vi "实时数据参数入列队.vi"(11 "发送实时数据选择框":T1) -> (0 "错误输出":errorcluster)   [LabVIEW 2016]
panel:
  out "数组":string[](array[string])
  # "水样测量"
  # "零点核查"
  # "跨度核查"
  # "加标回收"
  # "平行样"
  # "标样核查"
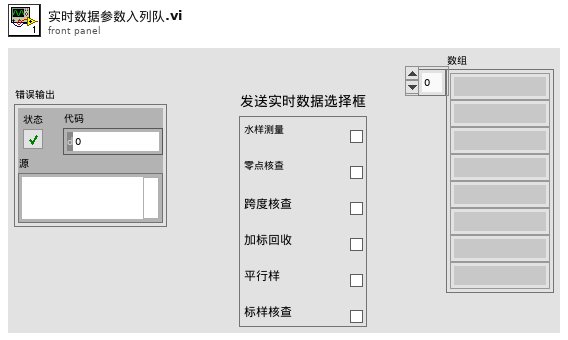
[diagram p1: front panel]
types:
  T1 = cluster{"水样测试":bool, "空白测试":bool, "跨度核查":bool, "加标回收":bool, "平行样":bool, "标样核查":bool}
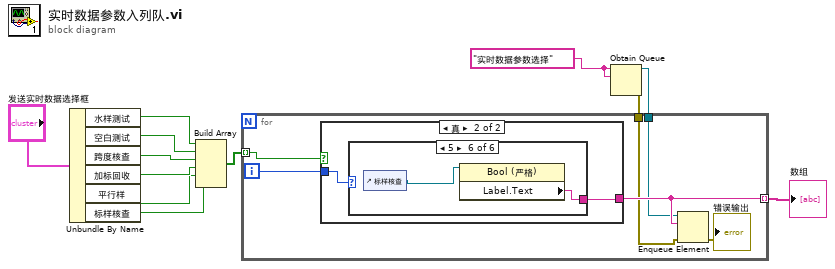
[diagram p0: block diagram]
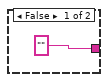
[diagram p2: hidden frame]
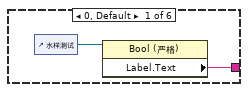
[diagram p3: hidden frame]
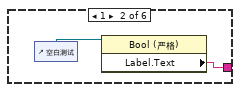
[diagram p4: hidden frame]
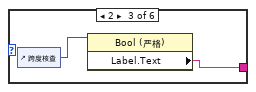
[diagram p5: hidden frame]
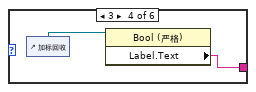
[diagram p6: hidden frame]
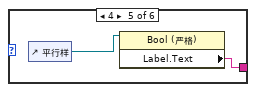
[diagram p7: hidden frame]
diagram:
  w3 = "实时数据参数选择" ("名称（未命名）")
  n1 = Unbundle By Name("发送实时数据选择框") -> ("水样测试"=w11:bool, "空白测试"=w10:bool, "跨度核查"=w9:bool, "加标回收"=w8:bool, "平行样"=w7:bool, "标样核查"=w1:bool)
  n2 = Build Array(w11, w10, w9, w8, w7, w1) -> (w6:bool[])
  n3 = Obtain Queue(name (unnamed)=w3, element data type=w3) -> (queue out=w4:refnum<queue>, error out=w2:errorcluster)  [unwired: 3 in, 1 out]
  n4 = for {
    tunnel: w6 -> [w18] mode=indexing
    tunnel: [w16] -> w5 mode=indexing
    tunnel: w4 -> [w15]
    tunnel: w2 -> [w14]
    i -> [w17]
    n5 = case shown="真" w18 {
      tunnel: w17 -> [_ w21]
      tunnel: ["" ("Label.Text") w20] -> w16
      frame False {
      }
      frame True {
        n6 = case shown="5" w21 {
          tunnel: [w22 w24 w27 w28 w30 w33] -> w20
          frame 0, Default {
            n7 = control-ref of="水样测试"() -> (w23:refnum<vi>)
            n8 = property class="Bool (严格)"(reference=w23) -> ("Label.Text"=w22:string)  [unwired: 1 in, 2 out]
          }
          frame 1 {
            n9 = control-ref of="空白测试"() -> (w25:refnum<vi>)
            n10 = property class="Bool (严格)"(reference=w25) -> ("Label.Text"=w24:string)  [unwired: 1 in, 2 out]
          }
          frame 2 {
            n11 = control-ref of="跨度核查"() -> (w26:refnum<vi>)
            n12 = property class="Bool (严格)"(reference=w26) -> ("Label.Text"=w27:string)  [unwired: 1 in, 2 out]
          }
          frame 3 {
            n13 = control-ref of="加标回收"() -> (w29:refnum<vi>)
            n14 = property class="Bool (严格)"(reference=w29) -> ("Label.Text"=w28:string)  [unwired: 1 in, 2 out]
          }
          frame 4 {
            n15 = control-ref of="平行样"() -> (w31:refnum<vi>)
            n16 = property class="Bool (严格)"(reference=w31) -> ("Label.Text"=w30:string)  [unwired: 1 in, 2 out]
          }
          frame 5 {
            n17 = control-ref of="标样核查"() -> (w32:refnum<vi>)
            n18 = property class="Bool (严格)"(reference=w32) -> ("Label.Text"=w33:string)  [unwired: 1 in, 2 out]
          }
        }
      }
    }
    n19 = Enqueue Element(queue=w15, element=w16, error in (no error)=w14) -> (error out=→"错误输出":errorcluster)  [unwired: 1 in, 2 out]
  }
  "数组" <- w5
